vi "interfejsRaspberryPi.vi"(11 "Error":errorcluster) -> ()   [LabVIEW 2014]
uses:
  interfejsVIs/AkcjaInterfejsu.ctl
  glownaMaszynaStanowVIs/AkcjaGFV.ctl
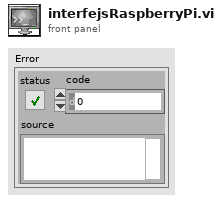
[diagram p1: front panel]
types:
  T1 = typedef "AkcjaInterfejsu.ctl" = enum16{"Polacz", "Wczytaj", "Zapisz", "Koniec"}
  T2 = enum16{"Standard", "Buffered", "CRLF", "Immediate"}
  T3 = typedef "AkcjaGFV.ctl" = enum16{"Czytaj", "Zapisz", "Reset"}
  T4 = typedef "WejsciaParametry.ctl" = cluster{"LEWO":bool, "PRAWO":bool, "GORA":bool, "DOL":bool, "Praca reczna":bool, "Stop":bool, "Start":bool, "Komora":bool, "Wyjscie":bool, "Rodzaj pomiarow":T5, "Czas pomiaru [s]":dbl, "Czas inicjalizacji ramion [s]":dbl, "Liczba punktów":i32, "Liczba płaszczyzn":i32, "Komora nadawcza":bool, "Komora odbiorcza":bool}
  T5 = typedef "RodzajPomiarow.ctl" = enum16{"Izolacyjność Akustyczna ISO 10140", "Losowanie punktów", "Sekwencja testowa"}
  T6 = typedef "WyjsciaParametry.ctl" = cluster{"Nad. lewo":bool, "Nad.  prawo":bool, "Nad.  gora":bool, "Nad. doł":bool, "Dzialanie":bool, "Pomiar":bool, "Odb. lewo":bool, "Odb.  prawo":bool, "Odb.  gora":bool, "Odb. dol":bool, "Pozostalo punktow":i32, "Nad. elewacja":i32, "Nad. azymut":i32, "Odb. elewacja":i32, "Odb. azymut":i32, "TCP Error":bool, "TCP Error Code":i32, "LINX Error":bool, "LINX Error Code":i32, "Nastepny elewacja":i32, "Nastepny azymut":i32, "Coords Error":bool, "Inicjalizacja pozycji":bool}
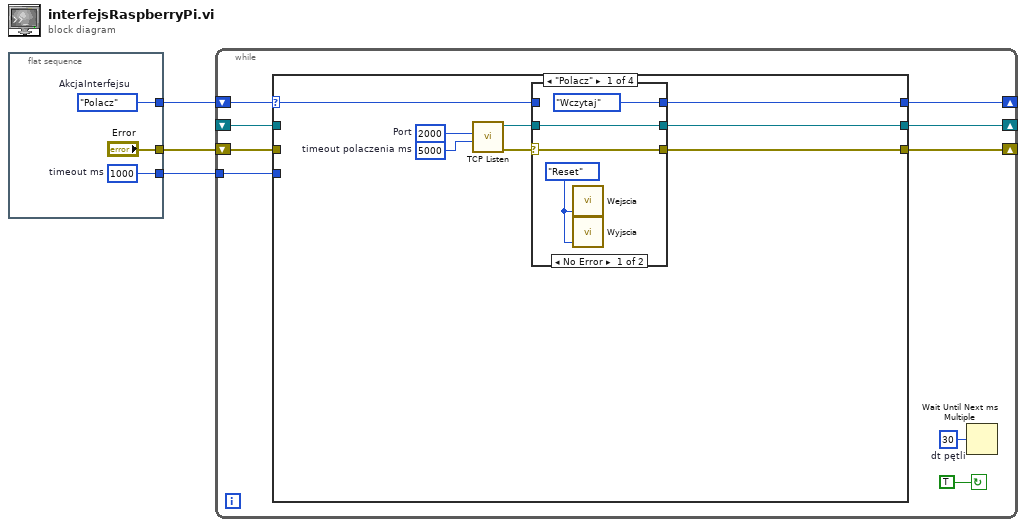
[diagram p0: block diagram]
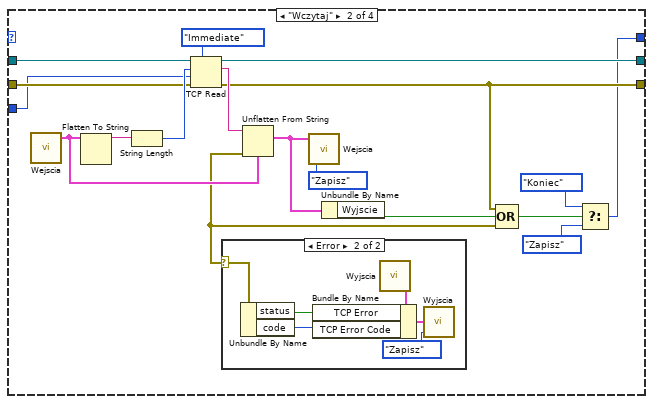
[diagram p3: hidden frame]
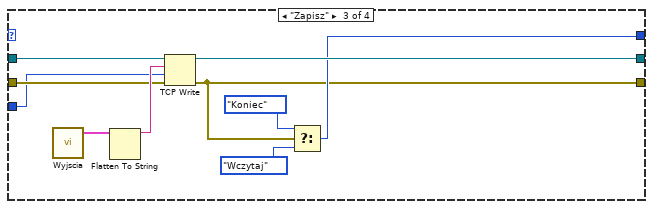
[diagram p5: hidden frame]
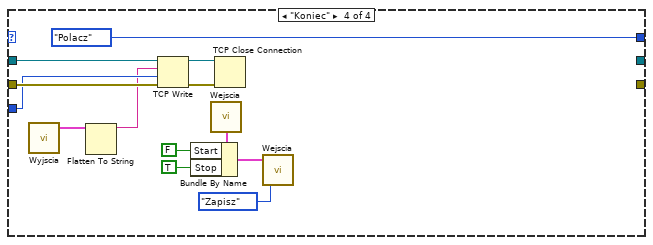
[diagram p6: hidden frame]
diagram:
  n1 = flat-sequence {
    tunnel: [w6] -> w3
    tunnel: [w5] -> w2
    tunnel: ["Error"] -> w1
    frame #0 {
      w5 = 1000  # timeout ms
      w6 = AkcjaInterfejsu."Polacz"  # AkcjaInterfejsu
    }
  }
  n2 = while {
    shift-right: [w14] -> _
    shift-left: w3 -> [w15]
    shift-right: [w13] -> _
    shift-left: _ -> [w11]
    shift-right: [w12] -> _
    shift-left: w1 -> [w10]
    tunnel: w2 -> [w8]
    stop <- TRUE continue-if-true
    w7 = u32 30  # dt pętli
    n3 = case shown="\"Polacz\"" w15 {
      selector: w15 -> [w20 _ _ _]
      tunnel: [w19 w32 w56 AkcjaInterfejsu."Polacz" ("f")] -> w14
      tunnel: [w18 w38 w60 _] -> w13
      tunnel: [w17 w36 w55 _] -> w12
      tunnel: w11 -> [_ w41 w63 w71]
      tunnel: w10 -> [_ w40 w62 w68]
      tunnel: w8 -> [_ w39 w61 w67]
      frame "Polacz" {
        w16 = 5000  # timeout polaczenia ms
        w23 = u16 2000  # Port
        n4 = call <vilib>:"TCP Listen.vi"("timeout ms (wait forever: -1)"=w16, "port"=w23) -> ("error out"=w22:errorcluster, "connection ID"=w21:refnum<k5>)  [unwired: 5 in, 3 out]
        n5 = case shown="No Error" w22 {
          selector: w22 -> [w27 w30]
          tunnel: w21 -> [w25 w29]
          tunnel: [w27 w30] -> w17
          tunnel: [AkcjaInterfejsu."Wczytaj" ("AkcjaInterfejsu") w28] -> w19
          tunnel: w20 -> [_ w28]
          tunnel: [w25 w29] -> w18
          frame No Error {
            w24 = AkcjaGFV."Reset" ("Akcja")
            n6 = call "Wejscia.vi"("Akcja"=w24) -> ()  [unwired: 4 in, 1 out]
            n7 = call "Wyjscia.vi"("Akcja"=w24) -> ()  [unwired: 4 in, 1 out]
          }
          frame Error {
          }
        }
      }
      frame "Wczytaj" {
        n8 = call "Wejscia.vi"() -> ("Wyjście"=w43:T4)  [unwired: 5 in]
        n9 = Flatten To String(anything=w43) -> (data string=w48:string)  [unwired: 3 in, 2 out]
        n10 = String Length(string=w48) -> (length=w47:i32)
        n11 = TCP Read(connection ID=w41, bytes to read=w47, error in (no error)=w40, 7:T2."Immediate" ("mode (standard)"), 9:w39) -> (connection ID out=w38:refnum<k5>, data out=w44:string, error out=w36:errorcluster)
        n12 = Unflatten From String(type=w43, binary string=w44) -> (value=w42:T4, error out=w31:errorcluster)  [unwired: 3 in, 1 out]
        n13 = case shown="Error" w31 {
          selector: w31 -> [_ w51]
          frame No Error {
          }
          frame Error {
            n14 = Unbundle By Name(w51) -> ("status"=w49:bool, "code"=w50:i32)
            n15 = call "Wyjscia.vi"() -> ("Wyjście"=w54:T6)  [unwired: 5 in]
            n16 = Bundle By Name(cluster=w54, "TCP Error"=w49, "TCP Error Code"=w50) -> (w53:T6)
            n17 = call "Wyjscia.vi"("Akcja"=AkcjaGFV."Zapisz", "Wejście"=w53) -> ()  [unwired: 3 in, 1 out]
          }
        }
        n18 = call "Wejscia.vi"("Akcja"=AkcjaGFV."Zapisz", "Wejście"=w42) -> ()  [unwired: 3 in, 1 out]
        n19 = Unbundle By Name(w42) -> ("Wyjscie"=w37:bool)
        n20 = Compound Arithmetic op=OR(w36, w37, w31) -> (w35:bool)
        n21 = Select(t=AkcjaInterfejsu."Koniec" ("AkcjaInterfejsu"), s=w35, f=AkcjaInterfejsu."Zapisz") -> (s? t:f=w32:T1)
      }
      frame "Zapisz" {
        n22 = call "Wyjscia.vi"() -> ("Wyjście"=w59:T6)  [unwired: 5 in]
        n23 = Flatten To String(anything=w59) -> (data string=w64:string)  [unwired: 3 in, 2 out]
        n24 = TCP Write(connection ID=w63, data in=w64, error in (no error)=w62, 9:w61) -> (connection ID out=w60:refnum<k5>, error out=w55:errorcluster)  [unwired: 1 out]
        n25 = Select(t=AkcjaInterfejsu."Koniec" ("AkcjaInterfejsu"), s=w55, f=AkcjaInterfejsu."Wczytaj") -> (s? t:f=w56:T1)
      }
      frame "Koniec" {
        n26 = call "Wyjscia.vi"() -> ("Wyjście"=w66:T6)  [unwired: 5 in]
        n27 = Flatten To String(anything=w66) -> (data string=w65:string)  [unwired: 3 in, 2 out]
        n28 = TCP Write(connection ID=w71, data in=w65, error in (no error)=w68, 9:w67) -> (connection ID out=w70:refnum<k5>, error out=w69:errorcluster)  [unwired: 1 out]
        n29 = call "Wejscia.vi"() -> ("Wyjście"=w73:T4)  [unwired: 5 in]
        n30 = Bundle By Name(cluster=w73, "Start"=FALSE, "Stop"=TRUE) -> (w75:T4)
        n31 = TCP Close Connection(connection ID=w70, error in (no error)=w69) -> ()  [unwired: 1 in, 2 out]
        n32 = call "Wejscia.vi"("Akcja"=AkcjaGFV."Zapisz", "Wejście"=w75) -> ()  [unwired: 3 in, 1 out]
      }
    }
    n33 = Wait Until Next ms Multiple(millisecond multiple=w7) -> ()  [unwired: 1 out]
  }
